vi "USB_CAN_RebuildCANID.vi"(1 "ExtFrame":bool, 3 "IDS":u8[](array[numeric])=[0, 0, 0, 0] format="%02x") -> (0 "ID":u32 format="%04x")   [LabVIEW 2011]
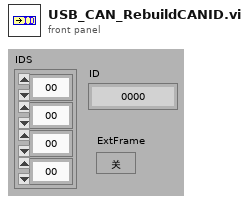
[diagram p1: front panel]
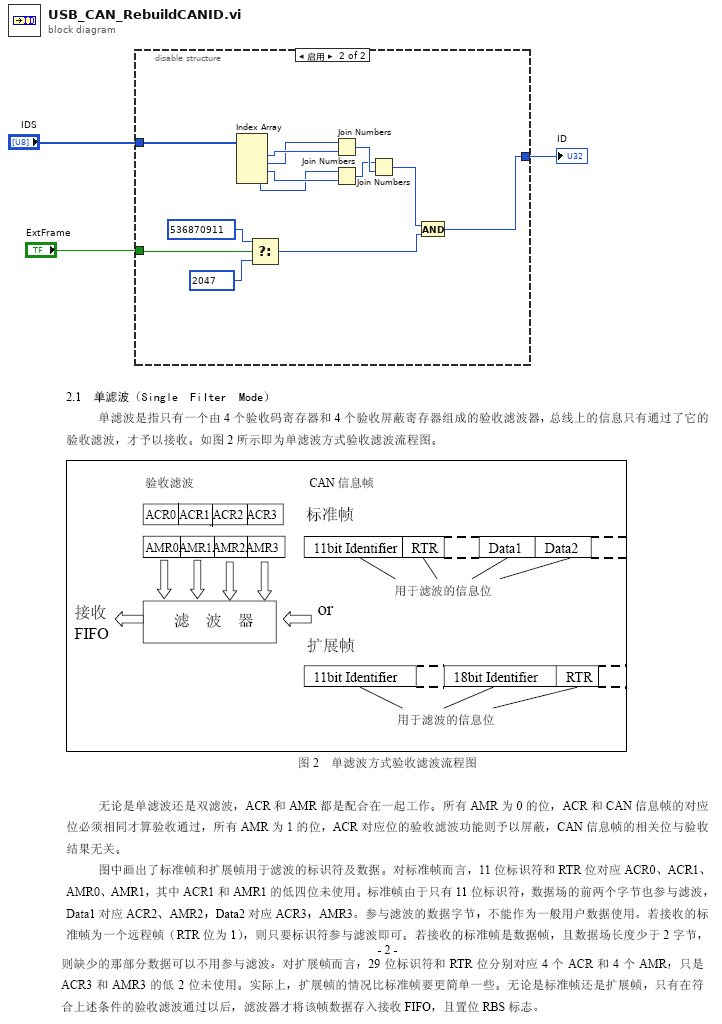
[diagram p0: block diagram]
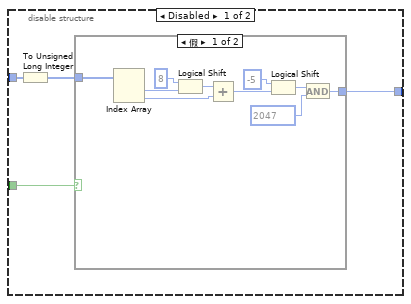
[diagram p2: hidden frame]
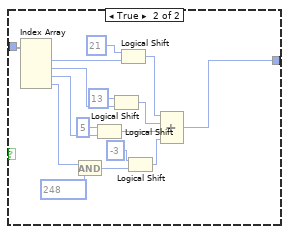
[diagram p3: hidden frame]
diagram:
  n1 = disable-structure shown="启用" {
    disable-tunnel: "IDS" -> [w7 w41]
    disable-tunnel: [w5 w42] -> w2
    disable-tunnel: "ExtFrame" -> [w4 w46]
    frame Disabled {
      n2 = To Unsigned Long Integer(number=w7) -> (unsigned 32bit integer=w6:u32[])
      n3 = case shown="假" w4 {
        tunnel: w6 -> [w16 w33]
        tunnel: [w8 w18] -> w5
        frame False {
          n4 = Index Array(array=w16) -> (element #1=w17:u32, element #2=w13:u32)  [unwired: 2 in]
          n5 = Logical Shift(y=i8 8, x=w17) -> (x << y=w14:u32)
          n6 = Add(x=w14, y=w13) -> (x+y=w12:u32)
          n7 = Logical Shift(y=i8 -5, x=w12) -> (x << y=w10:u32)
          n8 = And(x=w10, y=u32 2047) -> (x .and. y?=w8:u32)
        }
        frame True {
          n9 = Index Array(array=w33) -> (element #1=w27:u32, element #2=w29:u32, element #3=w21:u32, element #4=w31:u32)  [unwired: 4 in]
          n10 = And(x=w31, y=u32 248) -> (x .and. y?=w24:u32)
          n11 = Logical Shift(y=i8 5, x=w21) -> (x << y=w20:u32)
          n12 = Logical Shift(y=i8 13, x=w29) -> (x << y=w25:u32)
          n13 = Logical Shift(y=i8 21, x=w27) -> (x << y=w26:u32)
          n14 = Logical Shift(y=i8 -3, x=w24) -> (x << y=w22:u32)
          n15 = Compound Arithmetic op=ADD(w26, w25, w20, w22) -> (w18:u32)
        }
      }
    }
    frame Enabled {
      n16 = Index Array(array=w41) -> (element #1=w39:u8, element #2=w38:u8, element #3=w37:u8, element #4=w36:u8)  [unwired: 4 in]
      n17 = Select(t=u32 536870911 ("y"), s=w46, f=u32 2047 ("y")) -> (s? t:f=w43:u32)
      n18 = Join Numbers(hi=w38, lo=w39) -> ((hi.lo)=w35:u16)
      n19 = Join Numbers(hi=w36, lo=w37) -> ((hi.lo)=w34:u16)
      n20 = Join Numbers(hi=w34, lo=w35) -> ((hi.lo)=w40:u32)
      n21 = And(x=w40, y=w43) -> (x .and. y?=w42:u32)
    }
  }
  "ID" <- w2
